vi "FarFromTrajectory.vi"(10 "Path":dbl[][](array[numeric]), 11 "Position":dbl[](array[numeric])) -> (2 "Far from trajectory?":bool)   [LabVIEW 2018]
uses:
  <vilib>/Analysis/_algsub.llb/Real Vector Norm.vi
  <vilib>/Analysis/NI_AALPro.lvlib
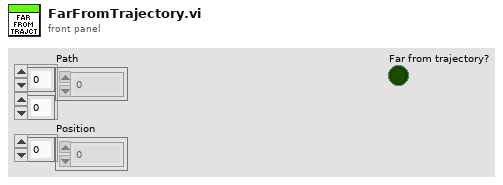
[diagram p1: front panel]
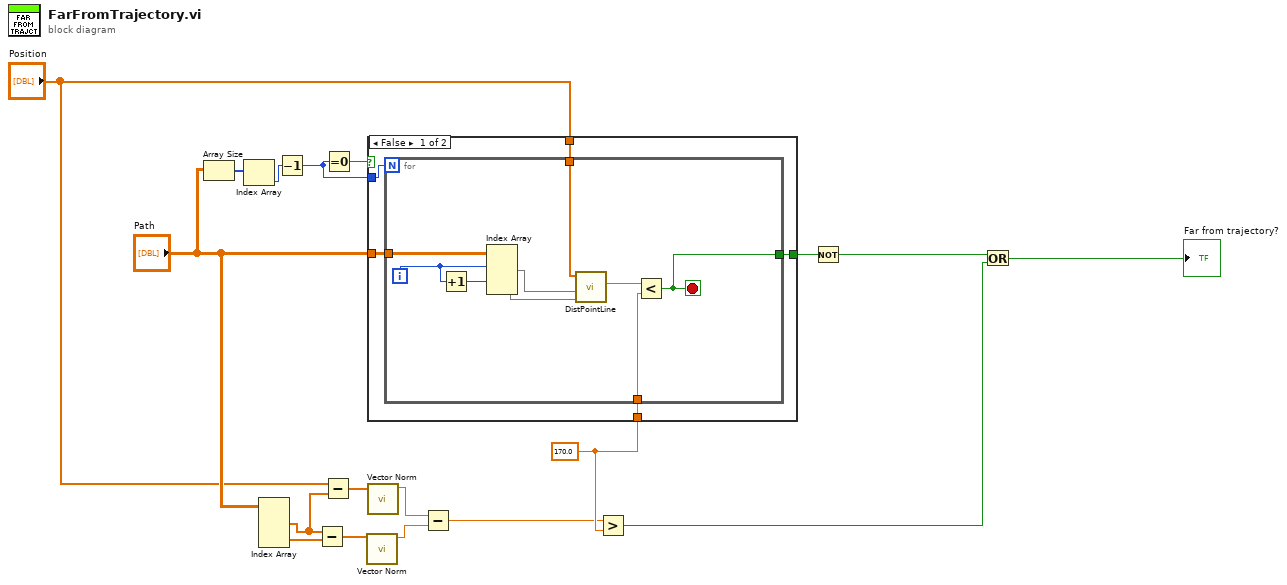
[diagram p0: block diagram]
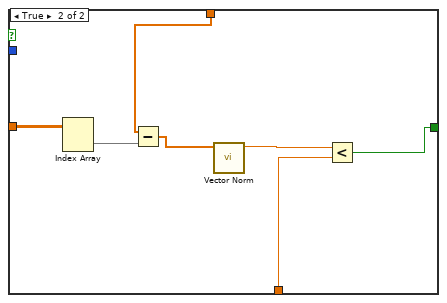
[diagram p2: hidden frame]
diagram:
  w7 = 170.0 ("y")
  n1 = Array Size(array="Path") -> (size(s)=w18:i32[])
  n2 = Index Array(array=w18) -> (element=w17:i32)  [unwired: 1 in]
  n3 = Index Array(array="Path") -> (element #1=w10:dbl[], element #2=w12:dbl[])  [unwired: 4 in]
  n4 = Decrement(x=w17) -> (x-1=w14:i32)
  n5 = Subtract(x=w10, y=w12) -> (x-y=w11:dbl[])
  n6 = Subtract(x="Position", y=w10) -> (x-y=w8:dbl[])
  n7 = Equal To 0?(x=w14) -> (x = 0?=w15:bool)
  n8 = call-poly <vilib>:"Vector Norm.vi"("Input Vector"=w11) -> ("norm"=w5:dbl)  [unwired: 9 in, 1 out]
  n9 = case shown="False" w15 {
    tunnel: "Path" -> [w23 w39]
    tunnel: "Position" -> [w22 w37]
    tunnel: [w21 w34] -> w16
    tunnel: w7 -> [w20 w33]
    tunnel: w14 -> [w19 _]
    frame False {
      n10 = for {
        N: w19 -> [_]
        tunnel: w23 -> [w32]
        tunnel: w22 -> [w27]
        tunnel: [w25] -> w21
        tunnel: w20 -> [w24]
        i -> [w30]
        stop <- w25 stop-if-true
        n11 = Increment(x=w30) -> (x+1=w31:i32)
        n12 = Index Array(array=w32, index (row) #1=w30, index (row) #2=w31) -> (element #1=w29:dbl[], element #2=w28:dbl[])  [unwired: 2 in]
        n13 = call "DistPointLine.vi"("P2"=w28, "P1"=w29, "Q"=w27) -> ("distance"=w26:dbl)  [unwired: 8 in]
        n14 = Less?(x=w26, y=w24) -> (x < y?=w25:bool)
      }
    }
    frame True {
      n15 = Index Array(array=w39) -> (element=w38:dbl[])  [unwired: 2 in]
      n16 = Subtract(x=w37, y=w38) -> (x-y=w36:dbl[])
      n17 = call-poly <vilib>:"Vector Norm.vi"("Input Vector"=w36) -> ("norm"=w35:dbl)  [unwired: 9 in, 1 out]
      n18 = Less?(x=w35, y=w33) -> (x < y?=w34:bool)
    }
  }
  n19 = call-poly <vilib>:"Vector Norm.vi"("Input Vector"=w8) -> ("norm"=w6:dbl)  [unwired: 9 in, 1 out]
  n20 = Subtract(x=w6, y=w5) -> (x-y=w4:dbl)
  n21 = Greater?(x=w4, y=w7) -> (0:w1:bool)
  n22 = Not(x=w16) -> (.not. x?=w3:bool)
  n23 = Or(x=w3, y=w1) -> (x .or. y?=→"Far from trajectory?":bool)
